vi "Acquisition_RawData.vi"() -> ()   [LabVIEW 2010]
uses:
  <vilib>/Utility/error.llb/DialogType.ctl
  <vilib>/DAQmx/read.llb/DAQmx Read (Analog 1D Wfm NChan NSamp).vi
  <vilib>/daqmx/miscellaneous.llb/DAQmx Fill In Error Info.vi
panel:
  in  "stop":bool
  out "Dur in Sec":i32
  in  "Feature Save To Path":path=path "E:/binTest.bin"
  out "EEG":waveform(dbl)(graph)
  out "EMG":waveform(dbl)(graph)
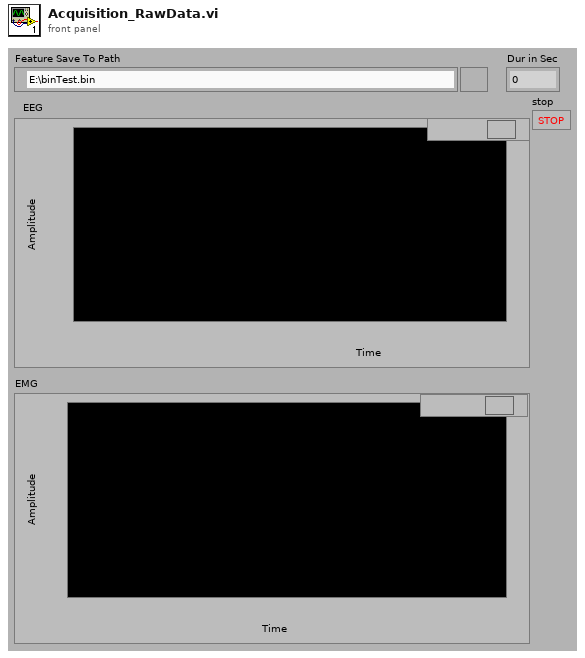
[diagram p1: front panel]
types:
  T1 = enum16{"open", "replace", "create", "open or create", "replace or create", "replace or create with confirmation"}
  T2 = typedef "DialogType.ctl" = u16
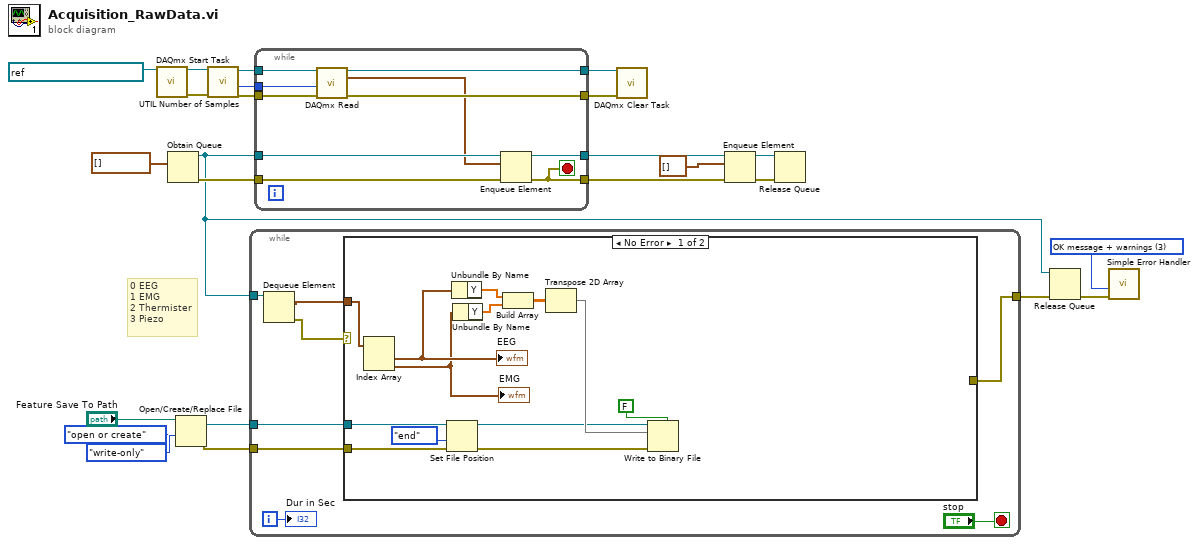
[diagram p0: block diagram]
diagram:
  w18 = T2 3 items=["no dialog", "OK message", "continue or stop message", "OK message + warnings", "continue/stop + warnings"] ("type of dialog (OK msg:1)")
  # "0 EEG\n1 EMG\n2 Thermister\n3 Piezo"
  n1 = call <vilib>:"DAQmx Start Task.vi"("task/channels in"=refnum<k21> "Thermal Acquisition") -> ("task out"=w14:refnum<k21>, "error out"=w13:errorcluster)  [unwired: 13 in]
  n2 = Obtain Queue(element data type=waveform(dbl)[] [] ("Measurement 2")) -> (queue out=w16:refnum<queue>, error out=w23:errorcluster)  [unwired: 4 in, 1 out]
  n3 = Open/Create/Replace File(file path (use dialog)="Feature Save To Path", operation (0:open)=T1."open or create", access (0:read/write)=enum16{"read/write", "read-only", "write-only"}."write-only") -> (refnum out=w2:refnum<file>, error out=w1:errorcluster)  [unwired: 3 in, 1 out]
  n4 = call "UTIL Number of Samples.vi"("Error In"=w13, "Task In"=w14) -> ("Error Out"=w9:errorcluster, "Samples/Chan"=w10:i32, "Task Out"=w11:refnum<k21>)  [unwired: 7 in]
  n5 = while {
    tunnel: w16 -> [w30]
    tunnel: [w29] -> w15
    tunnel: w2 -> [w26]
    tunnel: w1 -> [w25]
    i -> [w28]
    stop <- "stop" stop-if-true
    n6 = Dequeue Element(queue=w30) -> (element=w31:waveform(dbl)[], error out=w32:errorcluster)  [unwired: 2 in, 2 out]
    n7 = case shown="No Error" w32 {
      selector: w32 -> [_ w46]
      tunnel: w31 -> [w45 _]
      tunnel: [_ w46] -> w29
      tunnel: w26 -> [w36 _]
      tunnel: w25 -> [w35 _]
      frame No Error {
        n8 = Index Array(array=w45) -> (element #1=w44:waveform(dbl), element #2=w43:waveform(dbl))  [unwired: 2 in]
        "EMG" <- w43
        "EEG" <- w44
        n9 = Set File Position(refnum=w36, from (0:start)=enum16{"start", "end", "current"}."end", error in=w35) -> (refnum out=w33:refnum<file>, error out=w34:errorcluster)  [unwired: 1 in]
        n10 = Unbundle By Name(w44) -> ("Y"=w41:dbl[])
        n11 = Unbundle By Name(w43) -> ("Y"=w42:dbl[])
        n12 = Build Array(w41, w42) -> (w39:dbl[][])
        n13 = Transpose 2D Array(2D array=w39) -> (transposed array=w38:dbl[][])
        n14 = Write to Binary File(file (use dialog)=w33, data=w38, error in=w34, 5:FALSE ("prepend array or string size? (T)")) -> ()  [unwired: 2 in, 3 out]
      }
      frame Error {
      }
    }
    "Dur in Sec" <- w28
  }
  n15 = while {
    tunnel: [w56] -> w8
    tunnel: w16 -> [w55]
    tunnel: w23 -> [w54]
    tunnel: [w53] -> w22
    tunnel: [w52] -> w21
    tunnel: w11 -> [w51]
    tunnel: w10 -> [w50]
    tunnel: w9 -> [w49]
    tunnel: [w48] -> w7
    stop <- w52 stop-if-true
    n16 = call-poly <vilib>:"DAQmx Read.vi"("task/channels in"=w51, "number of samples per channel"=w50, "error in"=w49) -> ("task out"=w56:refnum<k21>, "data"=w47:waveform(dbl)[], "error out"=w48:errorcluster)  [unwired: 10 in]
    n17 = Enqueue Element(queue=w55, element=w47, error in (no error)=w54) -> (queue out=w53:refnum<queue>, error out=w52:errorcluster)  [unwired: 1 in, 1 out]
  }
  n18 = call <vilib>:"DAQmx Clear Task.vi"("task in"=w8, "error in"=w7) -> ()  [unwired: 13 in, 1 out]
  n19 = Enqueue Element(queue=w22, element=waveform(dbl)[] [] ("Measurement 2"), error in (no error)=w21) -> (queue out=w19:refnum<queue>, error out=w17:errorcluster)  [unwired: 1 in, 1 out]
  n20 = Release Queue(queue=w19, error in (no error)=w17) -> ()  [unwired: 1 in, 3 out]
  n21 = Release Queue(queue=w16, error in (no error)=w15) -> (error out=w6:errorcluster)  [unwired: 1 in, 2 out]
  n22 = call <vilib>:"Simple Error Handler.vi"("type of dialog (OK msg:1)"=w18, "error in (no error)"=w6) -> ()  [unwired: 3 in, 5 out]
